vi "Reset (SubVI).vi"(8 "error in (no error)":errorcluster, 11 "VISA Refnum in":refnum<visa-resource-name>) -> (0 "error out":errorcluster, 3 "VISA Refnum out":refnum<visa-resource-name>)   [LabVIEW 2023]
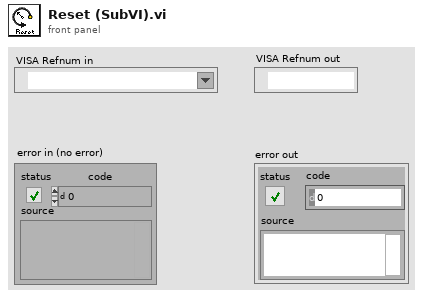
[diagram p1: front panel]
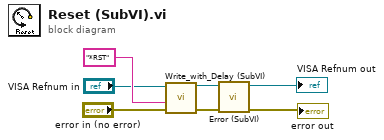
[diagram p0: block diagram]
diagram:
  n1 = call "Write_with_Delay (SubVI).vi"("error in (no error)"="error in (no error)", "Command"="*RST", "VISA Refnum in"="VISA Refnum in") -> ("error out"=w5:errorcluster, "VISA Refnum out"=w4:refnum<visa-resource-name>)  [unwired: 1 in]
  n2 = call "Error (SubVI).vi"("error in (no error)"=w5, "VISA Refnum in"=w4) -> ("error out"=→"error out":errorcluster, "VISA Refnum out"=→"VISA Refnum out":refnum<visa-resource-name>)  [unwired: 6 in, 2 out]
